vi "Fetch Multi Eval Meas List ES Flatness Subcarrier Index Current Results.vi"(6 "Range (Range 1)":T1=1 items=["Range 1"=1, "Range 2"=2], 8 "error in (no error)":errorcluster, 9 "Current Power (Minimum)":i32(ring) items=["Minimum", "Maximum"], 10 "Instance (1)":T2=1, 11 "VISA resource name":refnum<visa-resource-name>) -> (0 "error out":errorcluster, 1 "Results":i32[](array[numeric]), 2 "Reliability":i32, 3 "VISA resource name out":refnum<visa-resource-name>)   [LabVIEW 2020, in "Rohde&Schwarz CMWXP NR FR1 Measurement.lvlib"]
doc: "Return subcarrier indices of the equalizer spectrum flatness measurement for all measured list mode segments. At these SC indices, the current minimum or maximum power of the equalizer coefficients has been detected within the selected range.\n\nAttributes:\nRSCMWXPNRFR1M_ATTR_FETCH_MULTI_EVAL_MEAS_LIST_ES_FLATNESS_SUBCARRIER_INDEX_MINIMUM_CURRENT_RESULTS\nRSCMWXPNRFR1M_ATTR_FETCH_MULTI_EVAL_MEAS_LIST_ES_FLATNESS_SUBCARRIER_INDEX_MAXIMUM_CURRENT_RESULTS\n\nRemote-control commands:\nFETCh:NRSub:MEAS<i>:MEValuation:LIST:ESFLatness:SCINdex:MINimum<no>:CURRent?\nFETCh:NRSub:MEAS<i>:MEValuation:LIST:ESFLatness:SCINdex:MAXimum<no>:CURRent?"
uses:
  <instrlib>/Rohde&Schwarz CMWXP NR FR1 Measurement/Rohde&Schwarz CMWXP NR FR1 Measurement.lvlib
  <instrlib>/Rohde&Schwarz CMWXP NR FR1 Measurement/Private/_Instance.ctl
  <instrlib>/Rohde&Schwarz CMWXP NR FR1 Measurement/Private/_Range.ctl
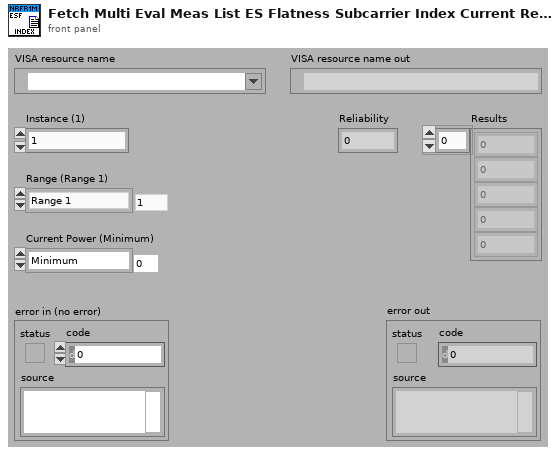
[diagram p1: front panel]
types:
  T1 = typedef "Rohde&Schwarz CMWXP NR FR1 Measurement.lvlib/_Range.ctl" = i32
  T2 = typedef "Rohde&Schwarz CMWXP NR FR1 Measurement.lvlib/_Instance.ctl" = i32
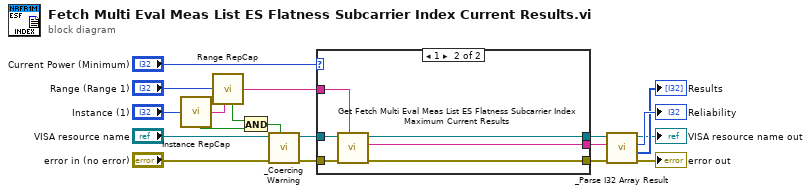
[diagram p0: block diagram]
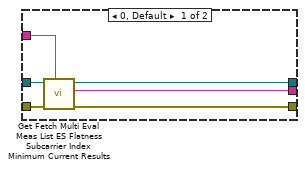
[diagram p2: hidden frame]
diagram:
  n1 = call <instrlib>:"Instance RepCap.vi"("Instance In"="Instance (1)") -> ("In Range?"=w14:bool, "RepCap Identifier Out"=w13:string)  [unwired: 1 in]
  n2 = call <instrlib>:"Range RepCap.vi"("Range In"="Range (Range 1)", "RepCap String In (\"\")"=w13) -> ("In Range?"=w12:bool, "RepCap Identifier Out"=w9:string)
  n3 = And(x=w12, y=w14) -> (x .and. y?=w17:bool)
  n4 = call <instrlib>:"_Coercing Warning.vi"("In Range?"=w17, "error in (no error)"="error in (no error)", "VISA resource name"="VISA resource name") -> ("error out"=w10:errorcluster, "VISA resource name out"=w11:refnum<visa-resource-name>)  [unwired: 7 in]
  n5 = case shown="1" "Current Power (Minimum)" {
    tunnel: w11 -> [w25 w31]
    tunnel: w10 -> [w24 w30]
    tunnel: w9 -> [w23 w29]
    tunnel: [w22 w28] -> w5
    tunnel: [w21 w27] -> w6
    tunnel: [w20 w26] -> w7
    frame 0, Default {
      n6 = call "Get Fetch Multi Eval Meas List ES Flatness Subcarrier Index Minimum Current Results"("Repeated Capabilities"=w23, "error in (no error)"=w24, "instrument handle"=w25) -> ("error out"=w20:errorcluster, "Fetch Multi Eval Meas List ES Flatness Subcarrier Index Minimum Current Results"=w21:string, "instrument handle out"=w22:refnum<visa-resource-name>)  [unwired: 6 in]
    }
    frame 1 {
      n7 = call "Get Fetch Multi Eval Meas List ES Flatness Subcarrier Index Maximum Current Results"("Repeated Capabilities"=w29, "error in (no error)"=w30, "instrument handle"=w31) -> ("error out"=w26:errorcluster, "Fetch Multi Eval Meas List ES Flatness Subcarrier Index Maximum Current Results"=w27:string, "instrument handle out"=w28:refnum<visa-resource-name>)  [unwired: 6 in]
    }
  }
  n8 = call <instrlib>:"_Parse I32 Array Result.vi"("error in (no error)"=w7, "Input String"=w6, "VISA resource name"=w5) -> ("error out"=→"error out":errorcluster, "Results"=→"Results":i32[], "Reliability"=→"Reliability":i32, "VISA resource name out"=→"VISA resource name out":refnum<visa-resource-name>)  [unwired: 5 in]
